vi "version.vi"(8 "error in (no error)":errorcluster, 11 "lv-builder-default in":refnum<class "lv-builder-default.lvclass">) -> (0 "error out":errorcluster, 3 "lv-builder-default out":refnum<class "lv-builder-default.lvclass">)   [LabVIEW 2015, in "lv-builder-default.lvclass"]
uses:
  lv-builder-default.lvclass
  _controls/configuration.ctl
  lv-builder/public/accessors/commit_hash_read.vi
  lv-builder-default.lvlib
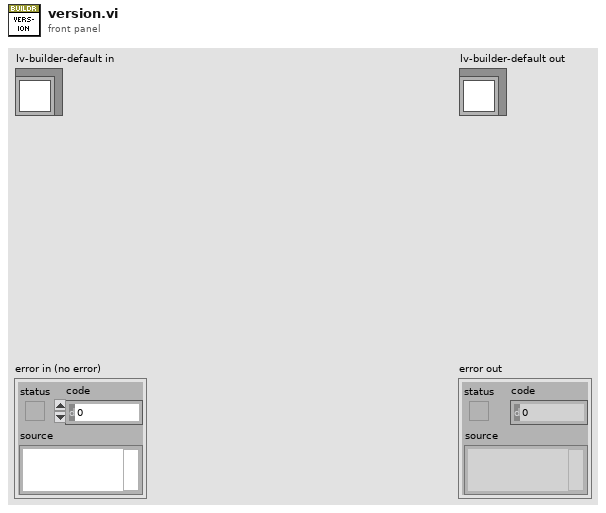
[diagram p1: front panel]
types:
  T1 = typedef "lv-builder-default.lvlib/configuration.ctl" = cluster{"project_file":string, "lvlibp_directory":string, "zip_directory":string, "lvlib_directory":string, "update_version_vi":string, "installer_post_file":string, "distribution_folder":string, "dependencies_folder":string, "bin_folder":string, "lvlib_post_action":u16, "installer_post_action":u16, "application_post_action":u16, "zip_post_action":u16}
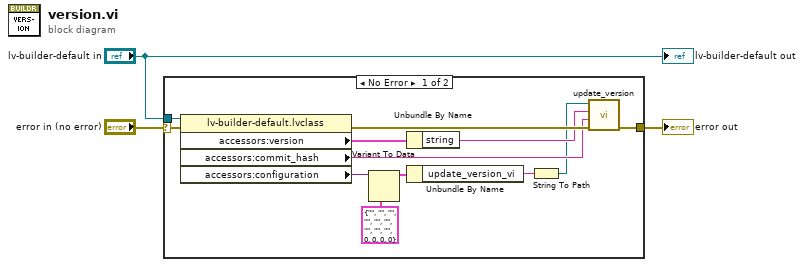
[diagram p0: block diagram]
diagram:
  n1 = case shown="No Error" "error in (no error)" {
    selector: "error in (no error)" -> [w15 w16]
    tunnel: [w5 w16] -> w2
    tunnel: "lv-builder-default in" -> [w14 _]
    frame No Error {
      n2 = property class="lv-builder-default.lvclass"(reference=w14, error in=w15) -> (error out=w10:errorcluster, "accessors:version"=w7:cluster{"variant":variant, "string":string}, "accessors:commit_hash"=w8:string, "accessors:configuration"=w13:variant)  [unwired: 1 out]
      n3 = Variant To Data(type=T1 {"project_file"="", "lvlibp_directory"="", "zip_directory"="", "lvlib_directory"="", "update_version_vi"="", "installer_post_file"="", "distribution_folder"="", "dependencies_folder"="", "bin_folder"="", "lvlib_post_action"=0, "installer_post_action"=0, "application_post_action"=0, "zip_post_action"=0} ("configuration"), Variant=w13) -> (data=w11:T1)  [unwired: 1 in, 1 out]
      n4 = Unbundle By Name(w7) -> ("string"=w6:string)
      n5 = Unbundle By Name(w11) -> ("update_version_vi"=w9:string)
      n6 = String To Path(string=w9) -> (path=w4:path)
      n7 = call "update_version.vi"("error in (no error)"=w10, "commit_hash"=w8, "version"=w6, "version_vi"=w4) -> ("error out"=w5:errorcluster)  [unwired: 7 in]
    }
    frame Error {
    }
  }
  "error out" <- w2
  "lv-builder-default out" <- "lv-builder-default in"
